vi "Get System Fonts.vi"(0 "Font IN":refnum<class "Font Class.lvclass">, 11 "error in (no error)":errorcluster) -> (4 "Font OUT":refnum<class "Font Class.lvclass">, 15 "error out":errorcluster)   [LabVIEW 2020, in "Exaprom PDF.lvlib" / "Font Class.lvclass"]
uses:
  <userlib>/labview-PDF-writer-master/LV Class/Fonts Class/Font Class.lvclass
  <userlib>/labview-PDF-writer-master/LV Class/Fonts Class/Font Class.lvclass/Font Class.ctl
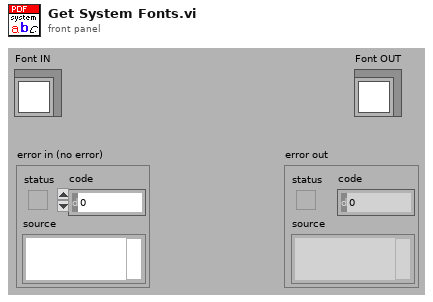
[diagram p1: front panel]
types:
  T1 = typedef "Exaprom PDF.lvlib/System Fonts.ctl" = cluster{"Font name [ ]":string[], "Font and file names [ ]":cluster{"Font name":string, "File name":string}[]}
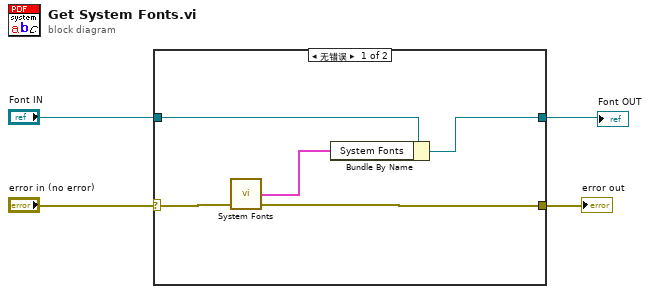
[diagram p0: block diagram]
diagram:
  n1 = case shown="无错误" "error in (no error)" {
    selector: "error in (no error)" -> [w7 w11]
    tunnel: [w5 w11] -> w3
    tunnel: [w9 w10] -> w2
    tunnel: "Font IN" -> [w8 w10]
    frame No Error {
      n2 = call <userlib>:"System Fonts.vi"("error in (no error)"=w7) -> ("error out"=w5:errorcluster, "System Fonts"=w6:T1)  [unwired: 3 in]
      n3 = Bundle By Name(cluster=w8, "System Fonts"=w6) -> (w9:refnum<class "Font Class.lvclass">)
    }
    frame Error {
    }
  }
  "error out" <- w3
  "Font OUT" <- w2
